vi "Set(array).vi"(8 "error in (no error)":errorcluster, 9 "value to set":refnum<class "JSON Value.lvclass">, 10 "Path Array":string[](array[string]), 11 "JSON Value in":refnum<class "JSON Value.lvclass">) -> (0 "error out":errorcluster, 3 "JSON Value out":refnum<class "JSON Value.lvclass">)   [LabVIEW 2016, in "JSON Value.lvclass"]
uses:
  JSON Value.lvclass
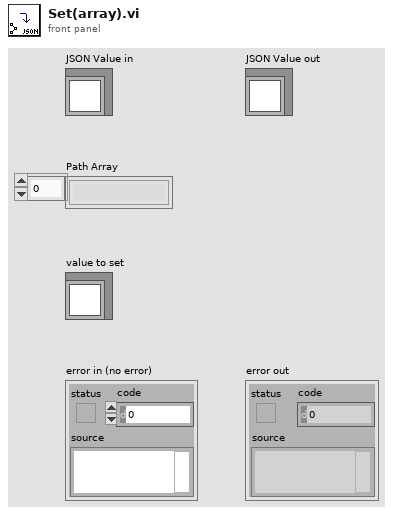
[diagram p1: front panel]
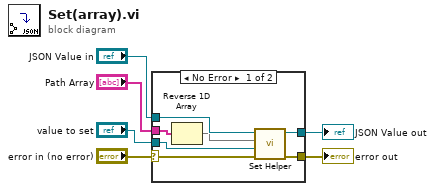
[diagram p0: block diagram]
diagram:
  n1 = case shown="No Error" "error in (no error)" {
    selector: "error in (no error)" -> [w11 w14]
    tunnel: [w9 w15] -> w4
    tunnel: "JSON Value in" -> [w12 w15]
    tunnel: "Path Array" -> [w13 _]
    tunnel: "value to set" -> [w7 _]
    tunnel: [w8 w14] -> w1
    frame No Error {
      n2 = Reverse 1D Array(array=w13) -> (reversed array=w10:string[])
      n3 = call "Set Helper.vi"("error in (no error)"=w11, "set value"=w7, "Array"=w10, "JSON Value in"=w12) -> ("error out"=w8:errorcluster, "JSON Value out"=w9:refnum<class "JSON Value.lvclass">)  [unwired: 6 in]
    }
    frame Error {
    }
  }
  "error out" <- w1
  "JSON Value out" <- w4
